vi "Stop Core.vi"(10 "final error code":i32, 11 "Command Processor in":refnum<class "Command Processor Actor.lvclass">) -> (3 "Command Processor out":refnum<class "Command Processor Actor.lvclass">)   [LabVIEW 2014, in "Robot Actor Framework.lvlib" / "Command Processor Actor.lvlib" / "Command Processor Actor.lvclass"]
doc: "(<B>Filename</B>: Actor Framework.lvlib:Actor.lvclass:Stop Core.vi)\n\nDefines what the actor does before it stops. Use the <B>final error code</B> input to determine whether the actor shut down in response to an error.\n\nBy default, this method does nothing. A descendant class may override it to define behavior, such as shutting down any processes the actor initiated in its override of the Actor Core method."
uses:
  Command Processor Actor.lvclass
  Command Processor Actor.lvclass/Command Processor Actor.ctl
  <vilib>/ActorFramework/Stop Msg/Stop Msg.lvclass/Stop Msg.ctl
  <vilib>/ActorFramework/Message Enqueuer/Message Enqueuer.lvclass/Message Enqueuer.ctl
  <vilib>/ActorFramework/Stop Msg/Send Emergency Stop.vi
  <vilib>/ActorFramework/Stop Msg/Send Normal Stop.vi
  <vilib>/ActorFramework/Message Enqueuer/Enqueue Critical.vi
  <vilib>/ActorFramework/Message Enqueuer/Enqueue.vi
  <vilib>/ActorFramework/Message Priority Queue/Priority Enqueue.vi
  <vilib>/ActorFramework/Stop Msg/Stop Msg.lvclass
  <vilib>/ni/Actors/State Actor/State Actor/State Actor.lvclass
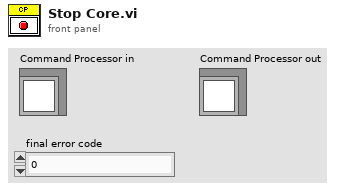
[diagram p1: front panel]
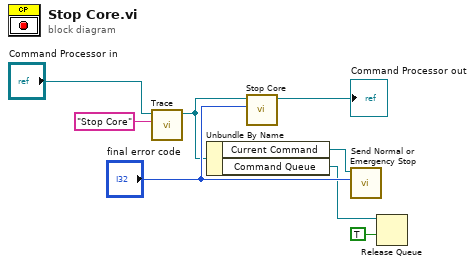
[diagram p0: block diagram]
diagram:
  n1 = call-dynamic "Trace.vi"("Command Processor Action"="Stop Core" ("Trace Message"), "Command Processor Actor in"="Command Processor in") -> ("Command Processor Actor out"=w2:refnum<class "Command Processor Actor.lvclass">)  [unwired: 8 in, 1 out]
  n2 = Unbundle By Name(w2) -> ("Current Command"=w7:refnum<class "Message Enqueuer.lvclass">, "Command Queue"=w5:refnum<queue>)
  n3 = call-parent "Stop Core.vi"("final error code"="final error code", "Actor in"=w2) -> ("Actor out"=→"Command Processor out":refnum<class "Command Processor Actor.lvclass">)  [unwired: 9 in]
  n4 = call <vilib>:"Send Normal or Emergency Stop.vi"("final error code"="final error code", "Message Enqueuer"=w7) -> ()  [unwired: 9 in, 1 out]
  n5 = Release Queue(queue=w5, force destroy? (F)=TRUE) -> ()  [unwired: 1 in, 3 out]
